vi "Set Global CSM Filter.vi"(10 "Group:CSM":string[](array[string]), 11 "GlobalLogFilter In":refnum<class "LogFilter.lvclass">) -> (3 "GlobalLogFilter Out":refnum<class "LogFilter.lvclass">)   [LabVIEW 2017, in "Communicable State Machine.lvlib" / "LogFilter.lvclass"]
doc: "### Set Global CSM Filter.vi\n\n-- <b>Controls</b> --\n- <b>Group:CSM</b>:\n- <b>GlobalLogFilter in</b>:\n\n-- <b>Indicators</b> --\n- <b>GlobalLogFilter out</b>:"
uses:
  LogFilter.lvclass
  LogFilter.lvclass/LogFilter.ctl
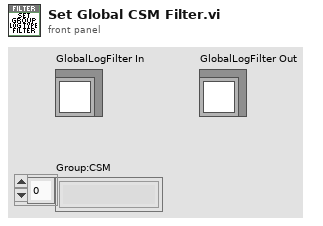
[diagram p1: front panel]
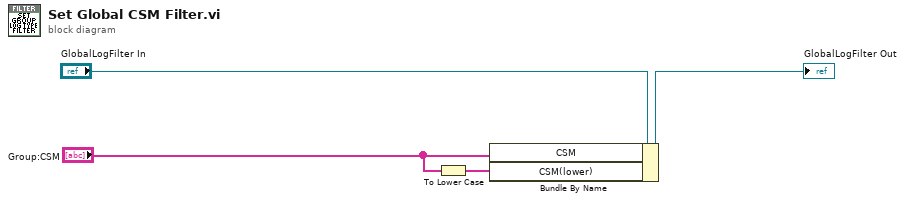
[diagram p0: block diagram]
diagram:
  n1 = To Lower Case(string="Group:CSM") -> (all lower case string=w1:string[])
  n2 = Bundle By Name(cluster="GlobalLogFilter In", "CSM"="Group:CSM", "CSM(lower)"=w1) -> (→"GlobalLogFilter Out":refnum<class "LogFilter.lvclass">)
